vi "write simulated ixon class.vi"(8 "error in (no error)":errorcluster, 10 "Sim_Ixon_Ultra.lvclass":refnum<class "Sim_Ixon_Ultra.lvclass">, 11 "SPARC4_Channel in":refnum<class "SPARC4_Channel.lvclass">) -> (0 "error out":errorcluster, 3 "SPARC4_Channel out":refnum<class "SPARC4_Channel.lvclass">)   [LabVIEW 2018, in "SPARC4_Channel.lvclass"]
uses:
  SPARC4_Channel.lvclass
  C:/Users/Denis/Desktop/S4ACS/S4ACS/Channel/Channel.lvclass
  Sim_Ixon_Ultra/Sim_Ixon_Ultra.lvclass
  C:/Users/Denis/Desktop/S4ACS/S4ACS/Sim_CCD/Sim_CCD.lvclass
  Sim_CCD/Sim_CCD.lvclass
  Channel/Channel.lvclass/Channel.ctl
  Channel/Channel.lvclass
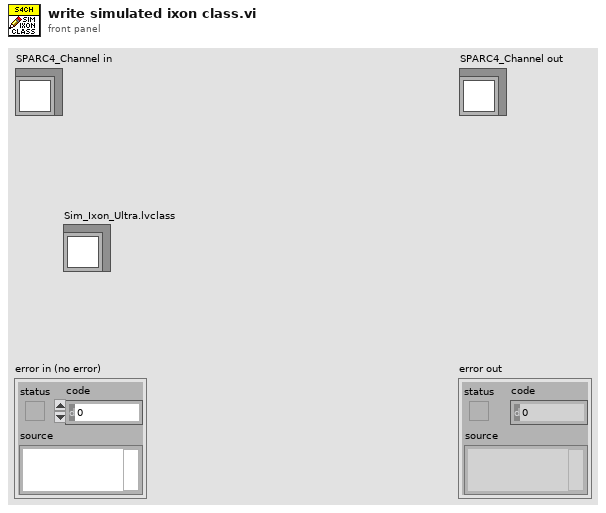
[diagram p1: front panel]
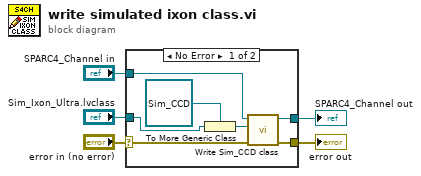
[diagram p0: block diagram]
diagram:
  n1 = case shown="No Error" "error in (no error)" {
    selector: "error in (no error)" -> [w10 w14]
    tunnel: [w9 w14] -> w4
    tunnel: [w11 w13] -> w2
    tunnel: "SPARC4_Channel in" -> [w12 w13]
    tunnel: "Sim_Ixon_Ultra.lvclass" -> [w8 _]
    frame No Error {
      n2 = To More Generic Class(target class=refnum<class "Sim_CCD.lvclass"> refnum ("Sim_CCD.lvclass"), reference=w8) -> (generic class reference=w6:refnum<class "Sim_CCD.lvclass">)
      n3 = call "Write Sim_CCD class.vi"("error in (no error)"=w10, "Sim_CCD.lvclass"=w6, "Channel in"=w12) -> ("error out"=w9:errorcluster, "Channel out"=w11:refnum<class "SPARC4_Channel.lvclass">)  [unwired: 7 in]
    }
    frame Error {
    }
  }
  "error out" <- w4
  "SPARC4_Channel out" <- w2
